vi "chart select.vi"(9 "difficulty":enum16{"easy", "hard"}(ring), 11 "song":enum16{"0", "1"}(ring)) -> (2 "file name":string)   [LabVIEW 2023]
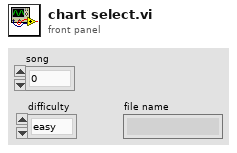
[diagram p1: front panel]
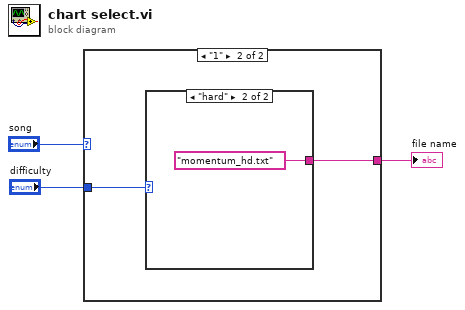
[diagram p0: block diagram]
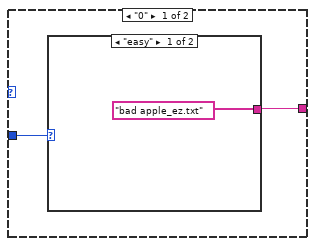
[diagram p2: hidden frame]
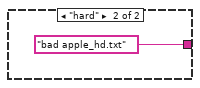
[diagram p3: hidden frame]
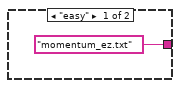
[diagram p4: hidden frame]
diagram:
  n1 = case shown="\"1\"" "song" {
    tunnel: [w5 w9] -> w3
    tunnel: "difficulty" -> [w4 w8]
    frame "0" {
      n2 = case shown="\"easy\"" w4 {
        tunnel: ["bad apple_ez.txt" "bad apple_hd.txt"] -> w5
        frame "easy" {
        }
        frame "hard" {
        }
      }
    }
    frame "1" {
      n3 = case shown="\"hard\"" w8 {
        tunnel: ["momentum_ez.txt" "momentum_hd.txt"] -> w9
        frame "easy" {
        }
        frame "hard" {
        }
      }
    }
  }
  "file name" <- w3
